vi "Tester_Create.vi"(0 "reference in":refnum<class "Tester.lvclass">, 1 "Reporter":refnum<class "Reporter.lvclass">, 5 "error in (no error)":errorcluster, 6 "LCR":refnum<class "BKP-891 LCR Meter.lvclass">, 8 "PSU":refnum<class "BKP-911x Power Supply.lvclass">, 10 "NI-DAQmx":refnum<class "NI-DAQmx.lvclass">) -> (13 "ProcessViRef":refnum<vi>, 14 "reference out":refnum<class "Tester.lvclass">, 19 "error out":errorcluster)   [LabVIEW 2018, in "Tester.lvclass"]
uses:
  Tester.lvclass
  BKP-891 LCR Meter_class/BKP-891 LCR Meter.lvclass
  BKP-911x Power Supply_class/BKP-911x Power Supply.lvclass
  NI-DAQmx_class/NI-DAQmx.lvclass
  Reporter_class/Reporter.lvclass
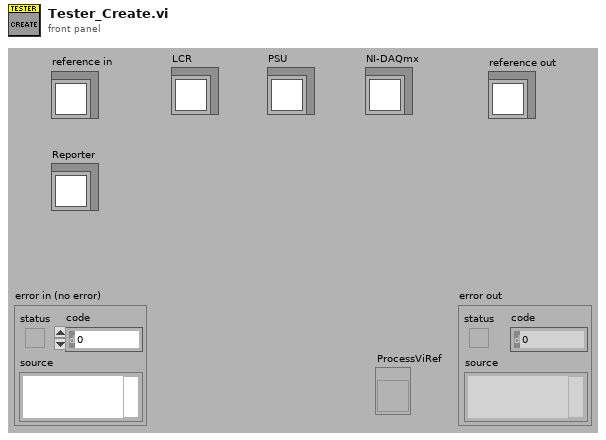
[diagram p1: front panel]
types:
  T1 = typedef "Tester.lvclass/ObjectAttributes.ctl" = cluster{"LCR":refnum<class "BKP-891 LCR Meter.lvclass">, "PSU":refnum<class "BKP-911x Power Supply.lvclass">, "NI-DAQmx":refnum<class "NI-DAQmx.lvclass">, "Reporter":refnum<class "Reporter.lvclass">, "Test Results":T2[]}
  T2 = typedef "Tester.lvclass/Test Result.ctl" = cluster{"Test Comment":string, "Signal Name":string, "Measured Value":dbl, "Upper Bound":dbl, "Lower Bound":dbl, "Pass?":bool}
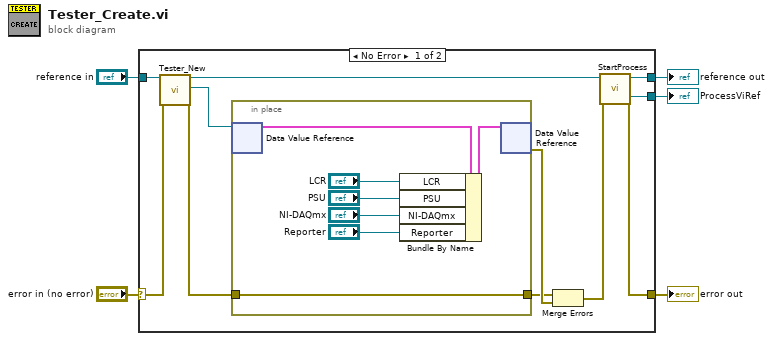
[diagram p0: block diagram]
diagram:
  n1 = case shown="No Error" "error in (no error)" {
    selector: "error in (no error)" -> [w15 w25]
    tunnel: [w7 w25] -> w4
    tunnel: "reference in" -> [w16 w24]
    tunnel: [w9 w24] -> w2
    tunnel: [w6 _] -> w1
    frame No Error {
      n2 = call "Tester_New.vi"("reference in"=w16, "error in (no error)"=w15) -> ("reference out"=w10:refnum<class "Tester.lvclass">, "DVRRefOut"=w13:refnum<data-value>, "error out"=w12:errorcluster)  [unwired: 14 in, 1 out]
      n3 = in-place {
        in-place-border: w12 -> [w21]
        in-place-border: [w21] -> w11
        n4 = in-place-dvr #1(w13) -> (w22:T1)  [unwired: 1 out]
        n5 = Bundle By Name(cluster=w22, "LCR"="LCR", "PSU"="PSU", "NI-DAQmx"="NI-DAQmx", "Reporter"="Reporter") -> (w23:T1)
        n6 = in-place-dvr #1(w23) -> (w14:errorcluster)  [unwired: 1 out]
      }
      n7 = Merge Errors(w11, w14) -> (w8:errorcluster)
      n8 = call "StartProcess.vi"("reference in"=w10, "error in (no error)"=w8) -> ("reference out"=w9:refnum<class "Tester.lvclass">, "ProcessViRef"=w6:refnum<vi>, "error out"=w7:errorcluster)  [unwired: 13 in, 2 out]
    }
    frame Error {
      # "VI-TechBaseTemplate_Simple_6x8x6"
    }
  }
  "error out" <- w4
  "reference out" <- w2
  "ProcessViRef" <- w1
